vi "Init-NetworkHandler.vi"(5 "Formatter.lvclass":refnum<class "Formatter.lvclass">, 7 "INetworkWriter":refnum<class "INetworkWriter.lvclass">, 8 "error in":errorcluster, 9 "Level":T1, 10 "Name":string, 11 "NetworkHandler in":refnum<class "StreamLogHandle.lvclass">) -> (0 "error out":errorcluster, 3 "NetworkHandler out":refnum<class "StreamLogHandle.lvclass">)   [LabVIEW 2024]
doc: "Initiates a new FileHandler-object with a name, log-level and a filepath for the log-file.\nThe handler processes LogRecords only if the level of the handler is greater or equal to the level of the LogRecord.\n\n____\nHAMPEL SOFTWARE ENGINEERING v2.2.2 (2025-01-16 15:41)"
uses:
  StreamLogHandle.lvclass/StreamLogHandle.ctl
  StreamLogHandle.lvclass
  <vilib>/Hampel Software Engineering/HSE Logger/LogLevel.ctl
  <vilib>/Hampel Software Engineering/HSE Logger/hse-logger.lvlib
  <vilib>/Hampel Software Engineering/HSE Logger/Formatter/Formatter.lvclass
  Stream/INetworkWriter/INetworkWriter.lvclass
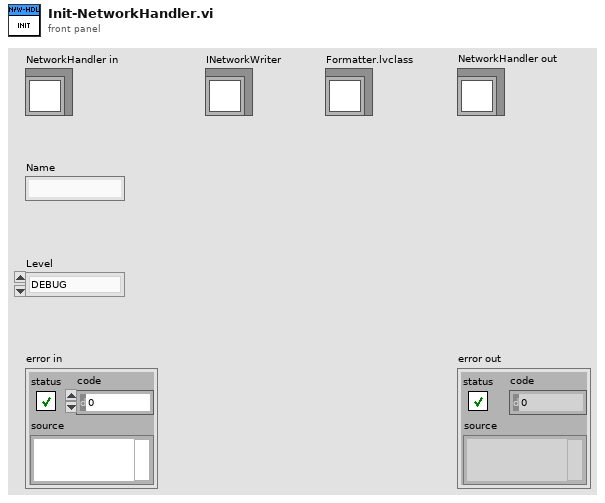
[diagram p1: front panel]
types:
  T1 = typedef "hse-logger.lvlib/LogLevel.ctl" = enum16{"DEBUG", "INFO", "WARNING", "ERROR", "CRITICAL"}
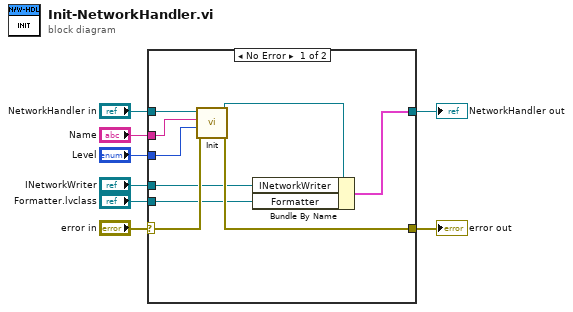
[diagram p0: block diagram]
diagram:
  n1 = case shown="No Error" "error in" {
    selector: "error in" -> [w17 w19]
    tunnel: [w11 w19] -> w7
    tunnel: [w16 w18] -> w6
    tunnel: "Name" -> [w15 _]
    tunnel: "Level" -> [w14 _]
    tunnel: "NetworkHandler in" -> [w13 w18]
    tunnel: "Formatter.lvclass" -> [w9 _]
    tunnel: "INetworkWriter" -> [w10 _]
    frame No Error {
      n2 = call-dynamic "Init.vi"("error in"=w17, "Level"=w14, "Name"=w15, "Handler"=w13) -> ("error out"=w11:errorcluster, "Handler out"=w12:refnum<class "NetworkHandler.lvclass">)  [unwired: 6 in]
      n3 = Bundle By Name(cluster=w12, "INetworkWriter"=w10, "Formatter"=w9) -> (w16:cluster{})
    }
    frame Error {
    }
  }
  "error out" <- w7
  "NetworkHandler out" <- w6
